vi "Auto_PID_Drive.vi"(8 "Tune_PID":bool, 9 "PID Turnin Gains":T1, 10 "Turning":dbl, 11 "Power":dbl) -> (2 "Turning":dbl, 3 "Power":dbl)   [LabVIEW 2014]
uses:
  General_VI/Global Var.vi
  <vilib>/addons/control/pid/pid.llb/PID (DBL).vi
  <vilib>/addons/control/pid/NI_PID_pid.lvlib
panel:
  out "Fault":bool
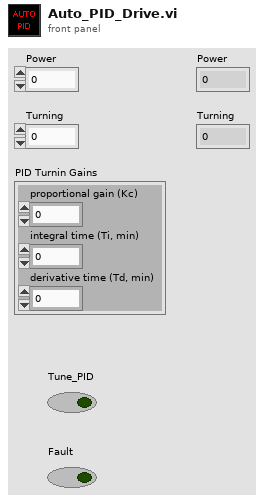
[diagram p1: front panel]
types:
  T1 = cluster{"proportional gain (Kc)":dbl, "integral time (Ti, min)":dbl, "derivative time (Td, min)":dbl}
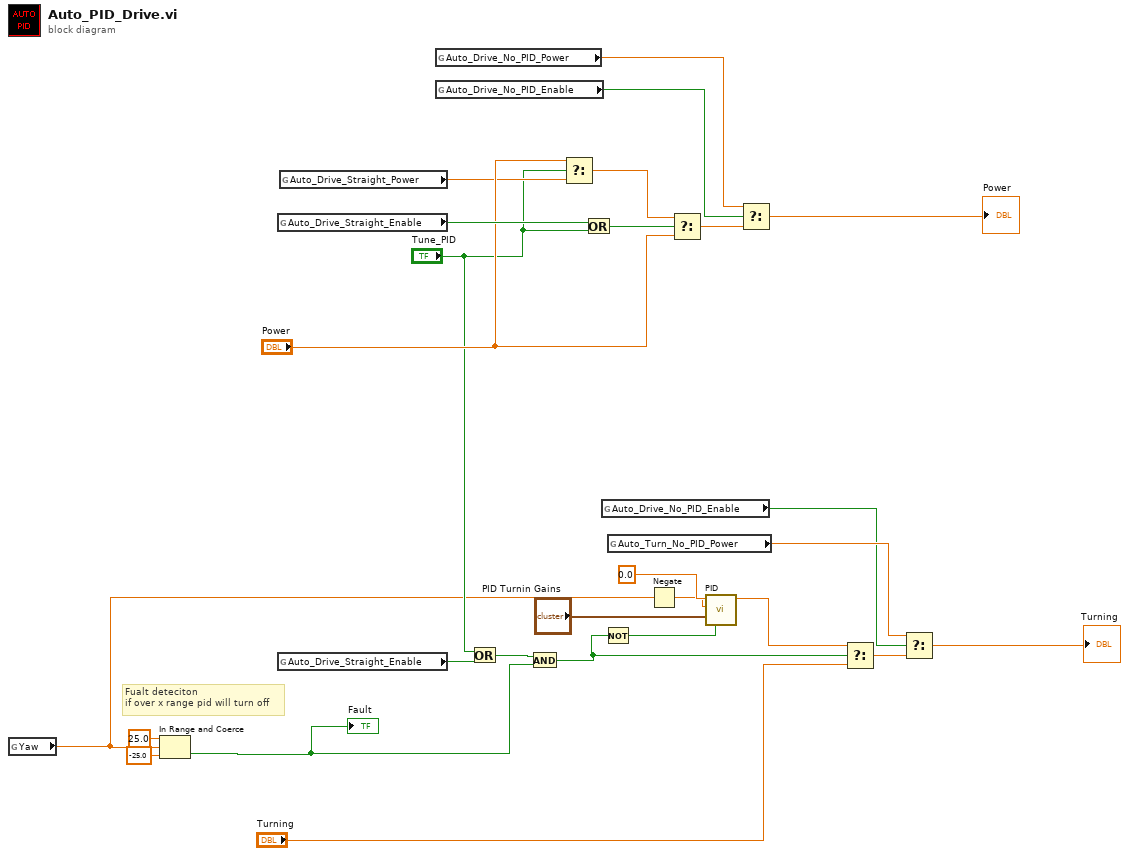
[diagram p0: block diagram]
diagram:
  # "Fualt deteciton \nif over x range pid will turn off"
  n1 = global read "Global Var.vi" "Yaw"() -> (w7:dbl)
  n2 = In Range and Coerce(upper limit=25.0, x=w7, lower limit=-25.0) -> (In Range?=w2:bool)  [unwired: 1 out]
  "Fault" <- w2
  n3 = global read "Global Var.vi" "Auto_Drive_Straight_Enable"() -> (w15:bool)
  n4 = global read "Global Var.vi" "Auto_Drive_Straight_Enable"() -> (w11:bool)
  n5 = global read "Global Var.vi" "Auto_Drive_Straight_Power"() -> (w13:dbl)
  n6 = global read "Global Var.vi" "Auto_Drive_No_PID_Power"() -> (w26:dbl)
  n7 = global read "Global Var.vi" "Auto_Drive_No_PID_Enable"() -> (w25:bool)
  n8 = Or(x="Tune_PID", y=w11) -> (x .or. y?=w3:bool)
  n9 = And(x=w3, y=w2) -> (x .and. y?=w1:bool)
  n10 = Select(t="Power", s="Tune_PID", f=w13) -> (s? t:f=w12:dbl)
  n11 = Or(x=w15, y="Tune_PID") -> (x .or. y?=w16:bool)
  n12 = global read "Global Var.vi" "Auto_Drive_No_PID_Enable"() -> (w4:bool)
  n13 = Not(x=w1) -> (.not. x?=w8:bool)
  n14 = global read "Global Var.vi" "Auto_Turn_No_PID_Power"() -> (w22:dbl)
  n15 = Negate(x=w7) -> (-x=w9:dbl)
  n16 = Select(t=w12, s=w16, f="Power") -> (s? t:f=w24:dbl)
  n17 = call-poly <vilib>:"PID.vi"("reinitialize? (F)"=w8, "PID gains"="PID Turnin Gains", "process variable"=w9, "setpoint"=0.0) -> ("output"=w18:dbl)  [unwired: 6 in, 1 out]
  n18 = Select(t=w26, s=w25, f=w24) -> (s? t:f=→"Power":dbl)
  n19 = Select(t=w18, s=w1, f="Turning") -> (s? t:f=w21:dbl)
  n20 = Select(t=w22, s=w4, f=w21) -> (s? t:f=→"Turning":dbl)
